vi "测试用.vi"() -> ()   [LabVIEW 2018]
uses:
  <vilib>/Utility/file.llb/Read Delimited Spreadsheet (DBL).vi
  <vilib>/express/express analysis/Spectral/Block/exnSpectralBlock spectral measurements RMS poly.vi
  <vilib>/express/express analysis/Spectral/Block/exnSpectralBlock spectral measurements RMS DDT.vi
  <vilib>/express/express analysis/Spectral/XNode/ExpressSpectralMeasurementsBlockNode.xnode
panel:
  in  "file path (dialog if empty) 2":path caption="文件路径 （空时为对话框）"
  in  "file path (dialog if empty)":path caption="文件路径 （空时为对话框）"
  out "Filtered Signal":dynamicdata(graph) caption="滤波后的信号"
  out "波形图 2":dynamicdata(graph)
  out "逐点滤波效果 2":dbl(graph)
  out "子数组":dbl[](array[numeric])
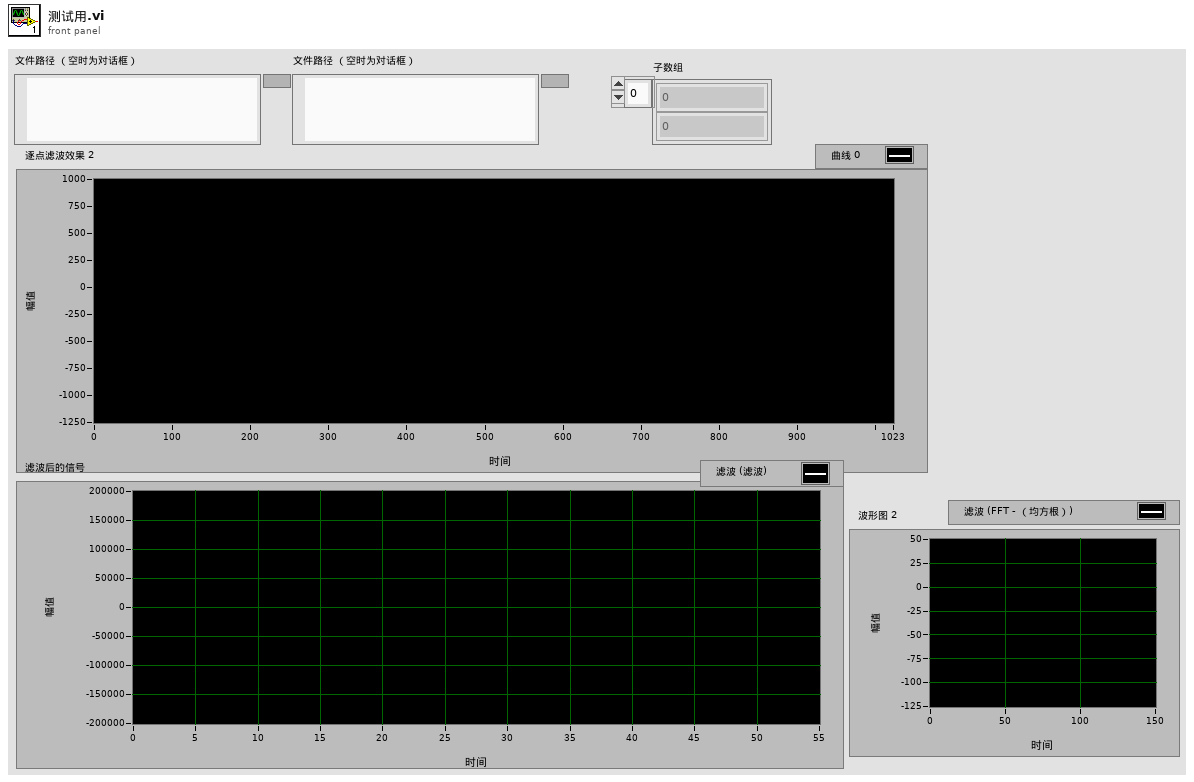
[diagram p1: front panel]
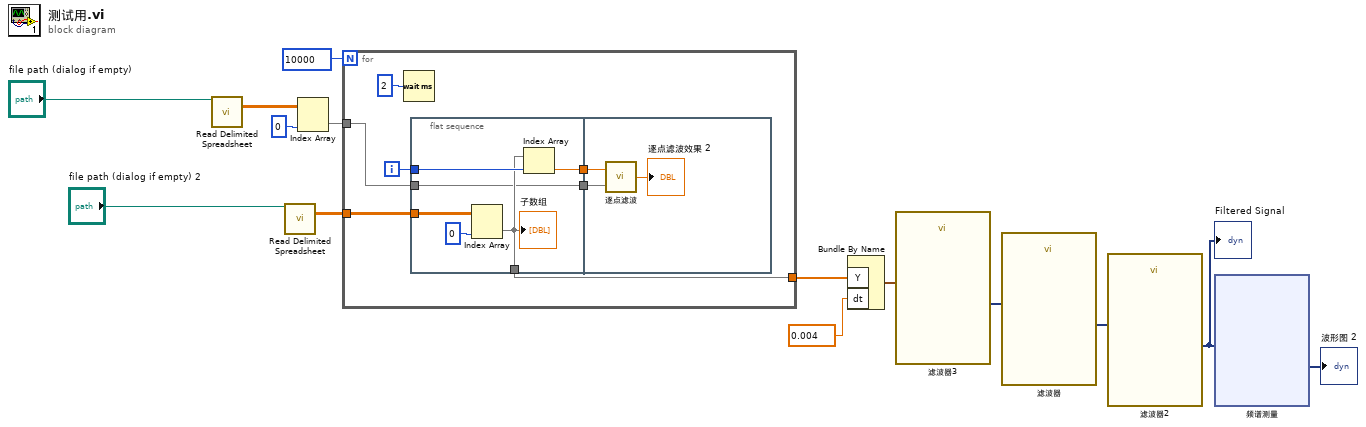
[diagram p0: block diagram]
diagram:
  n1 = call-poly <vilib>:"Read Delimited Spreadsheet.vi"("file path (dialog if empty)"="file path (dialog if empty)") -> ("all rows"=w3:dbl[][])  [unwired: 9 in, 5 out]
  n2 = call-poly <vilib>:"Read Delimited Spreadsheet.vi"("file path (dialog if empty)"="file path (dialog if empty) 2") -> ("all rows"=w13:dbl[][])  [unwired: 9 in, 5 out]
  n3 = Index Array(array=w3, index (col)=0 ("禁用的索引 (列)")) -> (element=w1:dbl[])  [unwired: 1 in]
  n4 = for {
    N: 10000 -> [_]
    tunnel: [w19] -> w8
    tunnel: w13 -> [w20]
    tunnel: w1 -> [w16]
    i -> [w21]
    n5 = Wait (ms)(milliseconds to wait=u32 2 ("等待时间（毫秒）")) -> ()  [unwired: 1 out]
    n6 = flat-sequence {
      tunnel: w21 -> [w27]
      tunnel: w20 -> [w26]
      tunnel: [w24] -> w19
      tunnel: [w23] -> w18
      tunnel: [w22] -> w17
      tunnel: w16 -> [w22]
      tunnel: w18 -> [w29]
      tunnel: w17 -> [w28]
      frame #0 {
        n7 = Index Array(array=w26, index (col)=0 ("禁用的索引 (列)")) -> (element=w24:dbl[])  [unwired: 1 in]
        "子数组" <- w24
        n8 = Index Array(array=w24, index=w27) -> (element=w23:dbl)
      }
      frame #1 {
        n9 = call "逐点滤波.vi"("Forward Coefficients"=w28, "输入x"=w29) -> ("Filtered x"=→"逐点滤波效果 2":dbl)
      }
    }
  }
  n10 = Bundle By Name("Y"=w8, "dt"=0.004) -> (w7:waveform(dbl))  [unwired: 1 in]
  n11 = call "滤波器3"("Signal"=w7) -> ("Filtered Signal"=w10:dynamicdata)  [unwired: 9 in, 1 out]
  n12 = call "滤波器"("Signal"=w10) -> ("Filtered Signal"=w9:dynamicdata)  [unwired: 9 in, 1 out]
  n13 = call "滤波器2"("Signal"=w9) -> ("Filtered Signal"=w6:dynamicdata)  [unwired: 9 in, 1 out]
  "Filtered Signal" <- w6
  n14 = xnode "频谱测量"("信号"=w6) -> ("测量输出"=→"波形图 2":dynamicdata)  [unwired: 1 in, 2 out]
